vi "Set Server State Ref.vi"(10 "Server Internal State Ref":refnum<data-value>, 11 "Template Server in":refnum<class "NW and PSD_server.lvclass">) -> (3 "Template Server out":refnum<class "NW and PSD_server.lvclass">)   [LabVIEW 2019, in "NW and PSD_server.lvlib" / "NW and PSD_server.lvclass"]
uses:
  NW and PSD_server.lvclass
  typeDefs/Server State Data.ctl
  NW and PSD_server.lvclass/NW and PSD_server.ctl
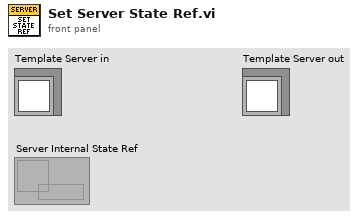
[diagram p1: front panel]
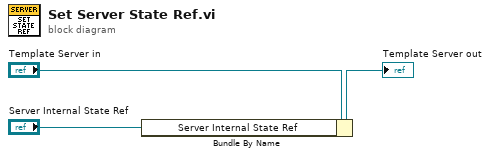
[diagram p0: block diagram]
diagram:
  n1 = Bundle By Name(cluster="Template Server in", "Server Internal State Ref"="Server Internal State Ref") -> (→"Template Server out":refnum<class "NW and PSD_server.lvclass">)
